vi "Set_RegData_String.vi"(8 "error in (no error)":errorcluster, 10 "string":string, 11 "Class in":refnum<class "IB_RegData_String.lvclass">) -> (0 "error out":errorcluster, 3 "Class out":refnum<class "IB_RegData_String.lvclass">)   [LabVIEW 2020, in "IB_RegData_String.lvclass"]
uses:
  <vilib>/AppBuilder/IB_Classes/RegData/RegData_String/IB_RegData_String.lvclass
  <vilib>/AppBuilder/IB_Classes/RegData/RegData_String/IB_RegData_String.lvclass/IB_RegData_String.ctl
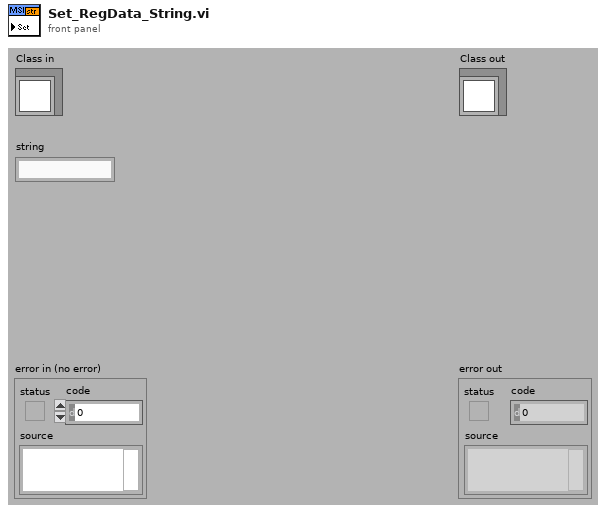
[diagram p1: front panel]
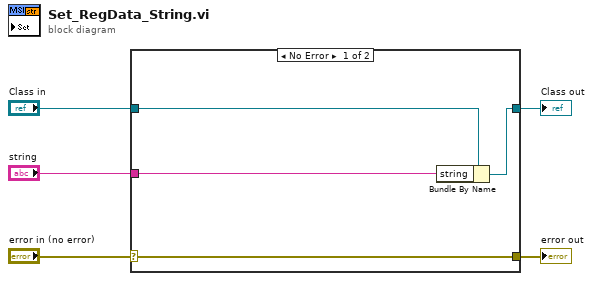
[diagram p0: block diagram]
diagram:
  n1 = case shown="No Error" "error in (no error)" {
    selector: "error in (no error)" -> [w9 w10]
    tunnel: [w9 w10] -> w4
    tunnel: [w7 w11] -> w2
    tunnel: "Class in" -> [w8 w11]
    tunnel: "string" -> [w6 _]
    frame No Error {
      n2 = Bundle By Name(cluster=w8, "string"=w6) -> (w7:refnum<class "IB_RegData_String.lvclass">)
    }
    frame Error {
    }
  }
  "error out" <- w4
  "Class out" <- w2
